vi "test.vi"(11 "data_in":cluster{"input":dbl}) -> (3 "data_out":cluster{"output":dbl})   [LabVIEW 2020]
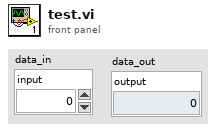
[diagram p1: front panel]
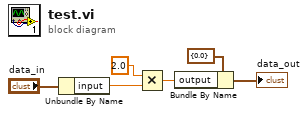
[diagram p0: block diagram]
diagram:
  n1 = Unbundle By Name("data_in") -> ("input"=w5:dbl)
  n2 = Multiply(x=2.0, y=w5) -> (x*y=w2:dbl)
  n3 = Bundle By Name(cluster=cluster{"output":dbl} {"output"=0.0} ("data_out"), "output"=w2) -> (→"data_out":cluster{"output":dbl})
